vi "Initialise Time Based Config.vi"(11 "Ship in":refnum<class "Ship.lvclass">) -> (3 "Ship out":refnum<class "Ship.lvclass">)   [LabVIEW 2021, in "Ship.lvclass"]
uses:
  Ship.lvclass
  Ship.lvclass/Ship.ctl
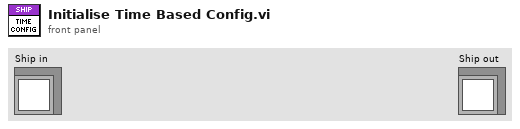
[diagram p1: front panel]
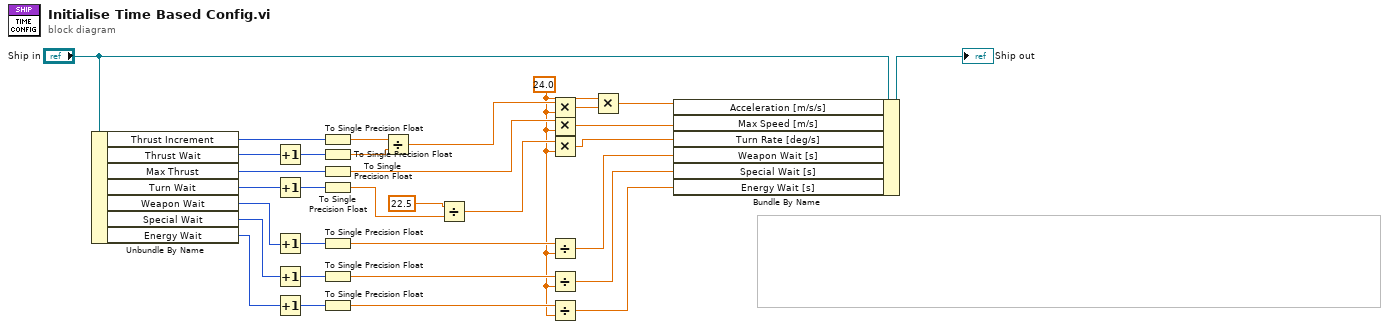
[diagram p0: block diagram]
diagram:
  w1 = sgl 24.0 ("y")
  n1 = Unbundle By Name("Ship in") -> ("Thrust Increment"=w26:i32, "Thrust Wait"=w30:i32, "Max Thrust"=w20:i32, "Turn Wait"=w27:i32, "Weapon Wait"=w13:i32, "Special Wait"=w11:i32, "Energy Wait"=w2:i32)
  n2 = Increment(x=w30) -> (x+1=w29:i32)
  n3 = Increment(x=w27) -> (x+1=w28:i32)
  n4 = Increment(x=w13) -> (x+1=w12:i32)
  n5 = Increment(x=w11) -> (x+1=w10:i32)
  n6 = Increment(x=w2) -> (x+1=w4:i32)
  n7 = To Single Precision Float(number=w26) -> (single precision float=w25:sgl)
  n8 = To Single Precision Float(number=w29) -> (single precision float=w24:sgl)
  n9 = To Single Precision Float(number=w20) -> (single precision float=w19:sgl)
  n10 = To Single Precision Float(number=w28) -> (single precision float=w22:sgl)
  n11 = To Single Precision Float(number=w12) -> (single precision float=w7:sgl)
  n12 = To Single Precision Float(number=w10) -> (single precision float=w9:sgl)
  n13 = To Single Precision Float(number=w4) -> (single precision float=w5:sgl)
  n14 = Divide(x=w25, y=w24) -> (x/y=w21:sgl)
  n15 = Divide(x=sgl 22.5, y=w22) -> (x/y=w17:sgl)
  n16 = Multiply(x=w21, y=w1) -> (x*y=w15:sgl)
  n17 = Multiply(x=w19, y=w1) -> (x*y=w18:sgl)
  n18 = Multiply(x=w17, y=w1) -> (x*y=w16:sgl)
  n19 = Divide(x=w7, y=w1) -> (x/y=w6:sgl)
  n20 = Divide(x=w9, y=w1) -> (x/y=w8:sgl)
  n21 = Divide(x=w5, y=w1) -> (x/y=w3:sgl)
  n22 = Multiply(x=w1, y=w15) -> (x*y=w14:sgl)
  n23 = Bundle By Name(cluster="Ship in", "Acceleration [m/s/s]"=w14, "Max Speed [m/s]"=w18, "Turn Rate [deg/s]"=w16, "Weapon Wait [s]"=w6, "Special Wait [s]"=w8, "Energy Wait [s]"=w3) -> (→"Ship out":refnum<class "Ship.lvclass">)
